vi "Copy Data Files.vi"(8 "error in":errorcluster, 10 "Data Files":cluster{"svg":path, "afm":path, "jpg":path}, 11 "Archivist in":refnum<class "Archivist.lvclass">) -> (0 "error out":errorcluster, 3 "Archivist out":refnum<class "Archivist.lvclass">)   [LabVIEW 2019, in "Archivist.lvclass"]
uses:
  Archivist.lvclass
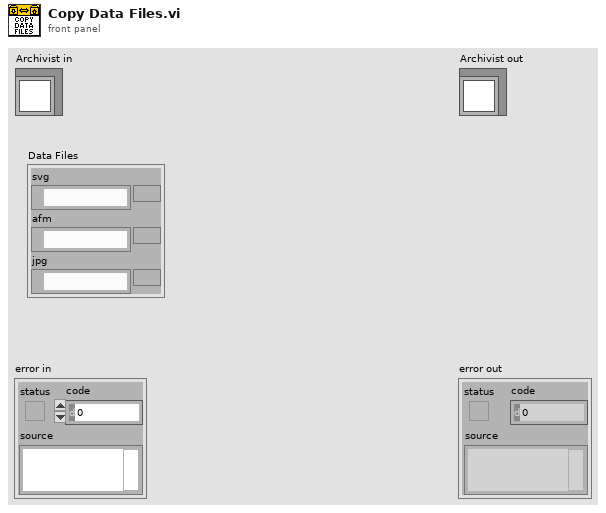
[diagram p1: front panel]
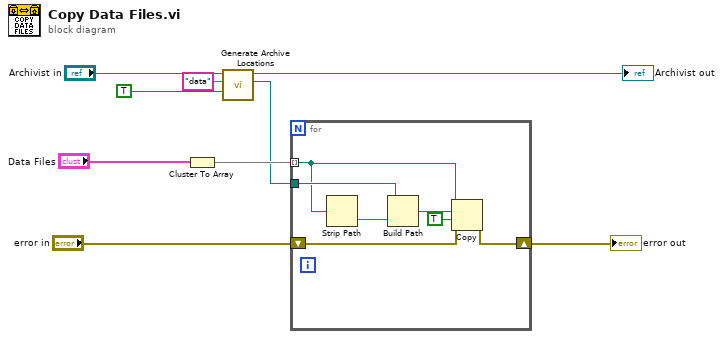
[diagram p0: block diagram]
diagram:
  n1 = Cluster To Array(cluster="Data Files") -> (array=w8:path[])
  n2 = call "Generate Archive Locations.vi"("Archive?"=TRUE, "Key"="data", "Archivist In"="Archivist in") -> ("Path Out"=w3:path, "Archivist Out"=→"Archivist out":refnum<class "Archivist.lvclass">)  [unwired: 7 in]
  n3 = for {
    tunnel: w3 -> [w12]
    tunnel: w8 -> [w11] mode=indexing
    shift-right: [w13] -> w7
    shift-left: "error in" -> [w14]
    n4 = Strip Path(path=w11) -> (name=w16:string)  [unwired: 1 out]
    n5 = Build Path(base path=w12, name or relative path=w16) -> (appended path=w15:path)
    n6 = Copy(8:w14, 9:TRUE ("overwrite (F)"), 10:w15, 11:w11) -> (0:w13:errorcluster)  [unwired: 1 in, 2 out]
  }
  "error out" <- w7
